vi "TCP Write Entire Buffer.vi"(8 "error in (no error)":errorcluster, 10 "data in":string, 11 "connection ID":refnum<k5>) -> (0 "error out":errorcluster, 2 "bytes written":i32, 3 "connection ID out":refnum<k5>)   [LabVIEW 2015, in "NI_InternetTK_Common_VIs.lvlib"]
doc: "Writes entire buffer to a TCP connection (retrying if a Time Out Error is returned)."
uses:
  NI_InternetTK_Common_VIs.lvlib
panel:
  in  "Num Retries":i32=10
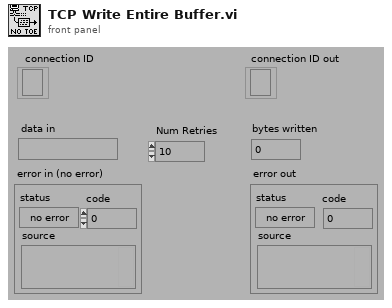
[diagram p1: front panel]
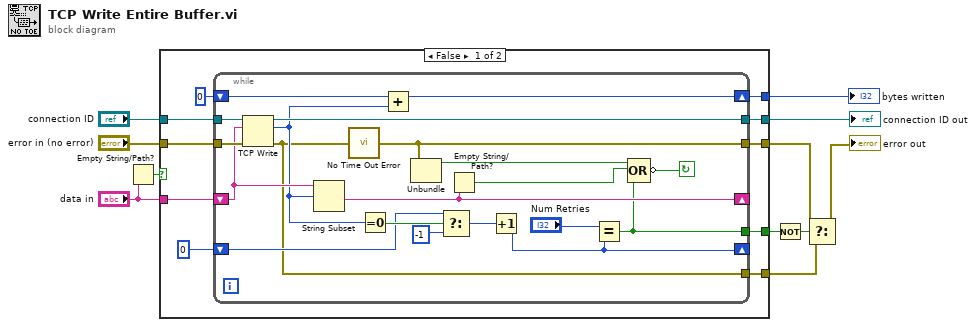
[diagram p0: block diagram]
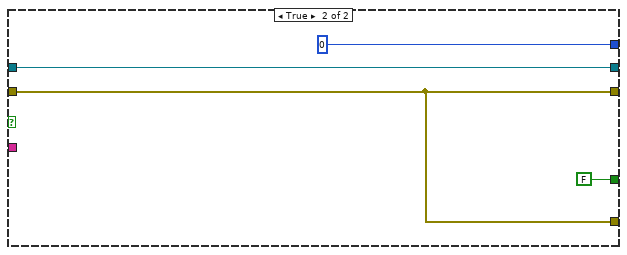
[diagram p2: hidden frame]
diagram:
  n1 = Empty String/Path?(string/path="data in") -> (empty?=w6:bool)
  n2 = case shown="False" w6 {
    tunnel: "data in" -> [w21 _]
    tunnel: [w20 0 ("y")] -> w8
    tunnel: [w18 w45] -> w9
    tunnel: [w17 w42] -> w1
    tunnel: "error in (no error)" -> [w16 w42]
    tunnel: "connection ID" -> [w15 w45]
    tunnel: [w13 FALSE] -> w4
    tunnel: [w12 w42] -> w3
    frame False {
      n3 = while {
        shift-left: 0 ("y") -> [w36]
        shift-right: [w35] -> w20
        tunnel: [w38] -> w18
        tunnel: [w34] -> w17
        shift-left: w21 -> [w39]
        shift-right: [w37] -> _
        tunnel: w16 -> [w40]
        tunnel: w15 -> [w41]
        shift-right: [w28] -> _
        shift-left: 0 -> [w30]
        tunnel: [w23] -> w13
        tunnel: [w22] -> w12
        stop <- w24 continue-if-true
        n4 = TCP Write(connection ID=w41, data in=w39, error in (no error)=w40) -> (connection ID out=w38:refnum<k5>, bytes written=w33:i32, error out=w22:errorcluster)  [unwired: 1 out]
        n5 = String Subset(string=w39, offset (0)=w33) -> (substring=w37:string)  [unwired: 1 out]
        n6 = call "No Time Out Error.vi"("error in (no error)"=w22) -> ("error out"=w34:errorcluster)  [unwired: 14 out]
        n7 = Equal To 0?(x=w33) -> (x = 0?=w32:bool)
        n8 = Add(x=w36, y=w33) -> (x+y=w35:i32)
        n9 = Unbundle(w34) -> ("status"=w26:bool)  [unwired: 2 out]
        n10 = Select(t=w30, s=w32, f=-1) -> (s? t:f=w29:i32)
        n11 = Empty String/Path?(string/path=w37) -> (empty?=w25:bool)
        n12 = Increment(x=w29) -> (x+1=w28:i32)
        n13 = Equal?(x="Num Retries", y=w28) -> (x = y?=w23:bool)
        n14 = Compound Arithmetic op=OR(w26, w25, w23) -> (invert w24:bool)
      }
    }
    frame True {
    }
  }
  "connection ID out" <- w9
  "bytes written" <- w8
  n15 = Not(x=w4) -> (.not. x?=w5:bool)
  n16 = Select(t=w1, s=w5, f=w3) -> (s? t:f=→"error out":errorcluster)
